vi "Connect Merge Error Terminals.vi"(8 "error in (no error)":errorcluster, 11 "DVR VI Path":path=path "D:/GitHub/LabVIEW/SLL/Tools/Class DVR API Generator/Test/Test VI.vi") -> (0 "error out":errorcluster)   [LabVIEW 2016, in "SLL Scripting.lvlib" / "SLL Class DVR API Generator.lvlib"]
uses:
  SLL Class DVR API Generator.lvlib
  <vilib>/Utility/traverseref.llb/TRef TravTarget.ctl
  <vilib>/Utility/traverseref.llb/VI Scripting - Traverse.lvlib
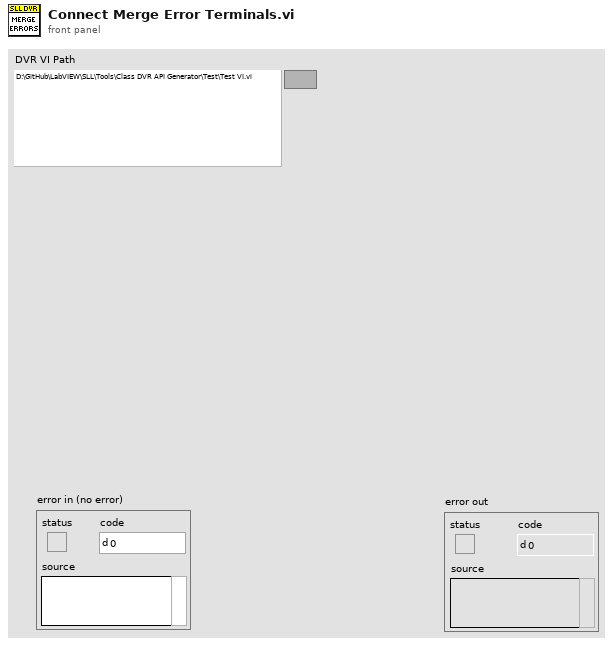
[diagram p1: front panel]
types:
  T1 = typedef "TRef TravTarget.ctl" = enum16{"FP", "BD", "Other"}
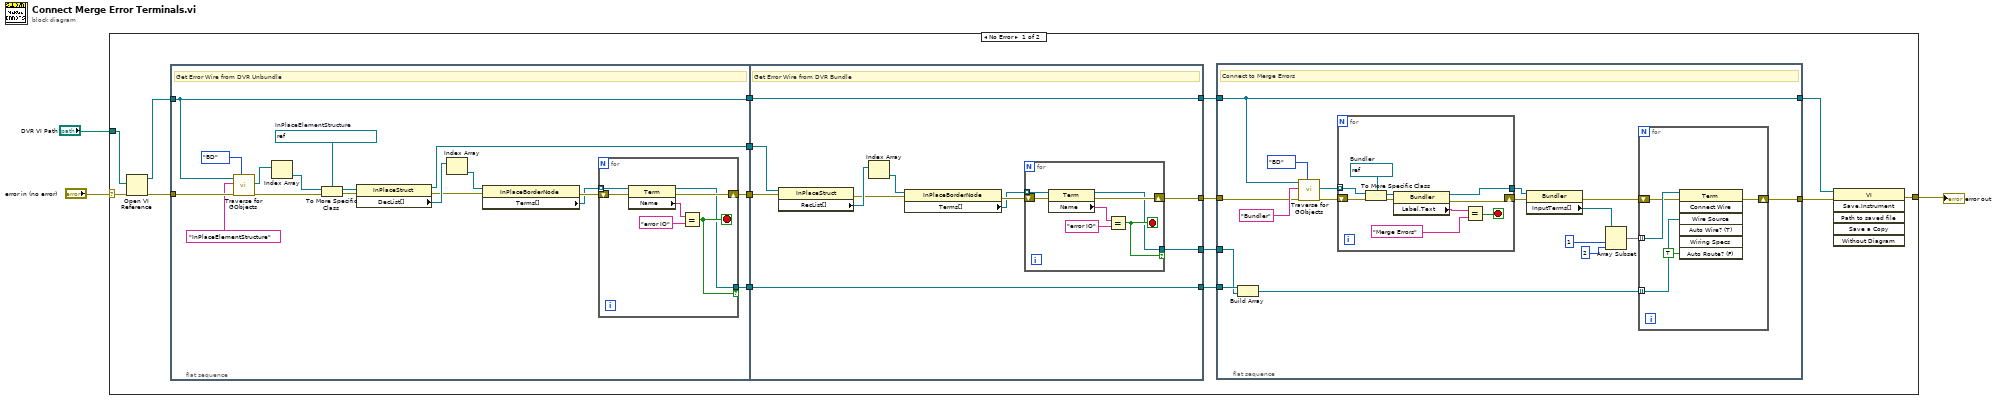
[diagram p0: block diagram]
diagram:
  n1 = case shown="No Error" "error in (no error)" {
    selector: "error in (no error)" -> [w18 w94]
    tunnel: [w16 w94] -> w2
    tunnel: "DVR VI Path" -> [w17 _]
    frame No Error {
      n2 = Open VI Reference(vi path=w17, error in (no error)=w18) -> (vi reference=w15:refnum<vi>, error out=w14:errorcluster)  [unwired: 4 in]
      n3 = flat-sequence {
        tunnel: w14 -> [w68]
        tunnel: w15 -> [w67]
        tunnel: [w67] -> w10
        tunnel: [w61] -> w9
        tunnel: [w60] -> w8
        tunnel: [w59] -> w7
        tunnel: [w86] -> w13
        tunnel: w10 -> [w86]
        tunnel: w9 -> [w82]
        tunnel: w8 -> [w81]
        tunnel: w7 -> [w80]
        tunnel: [w80] -> w6
        tunnel: [w77] -> w5
        tunnel: [w76] -> w4
        frame #0 {
          w53 = refnum<vi> refnum  # InPlaceElementStructure
          # "Get Error Wire from DVR Unbundle"
          n4 = call <vilib>:"Traverse for GObjects.vi"("Traverse Target"=TRef_TravTarget."BD", "error in (no error)"=w68, "Class Name"="InPlaceElementStructure", "VI Refnum"=w67) -> ("error out"=w55:errorcluster, "References"=w56:refnum<vi>[])  [unwired: 4 in, 2 out]
          n5 = Index Array(array=w56) -> (element=w54:refnum<vi>)  [unwired: 1 in]
          n6 = To More Specific Class(target class=w53, reference=w54, error in=w55) -> (specific class reference=w52:refnum<vi>, error out=w51:errorcluster)
          n7 = property class="InPlaceStruct"(reference=w52, error in=w51) -> (reference out=w60:refnum<vi>, error out=w64:errorcluster, "DecList[]"=w66:refnum<vi>[])
          n8 = Index Array(array=w66) -> (element=w65:refnum<vi>)  [unwired: 1 in]
          n9 = property class="InPlaceBorderNode"(reference=w65, error in=w64) -> (error out=w63:errorcluster, "Terms[]"=w62:refnum<vi>[])  [unwired: 1 out]
          n10 = for {
            tunnel: w62 -> [w75] mode=indexing
            shift-right: [w70] -> w61
            shift-left: w63 -> [w74]
            tunnel: [w69] -> w59 if=w71
            stop <- w71 stop-if-true
            n11 = property class="Term"(reference=w75, error in=w74) -> (reference out=w69:refnum<vi>, error out=w70:errorcluster, "Name"=w73:string)
            n12 = Equal?(x=w73, y="error IO") -> (x = y?=w71:bool)
          }
        }
        frame #1 {
          # "Get Error Wire from DVR Bundle"
          n13 = property class="InPlaceStruct"(reference=w81, error in=w82) -> (error out=w83:errorcluster, "RecList[]"=w85:refnum<vi>[])  [unwired: 1 out]
          n14 = Index Array(array=w85) -> (element=w84:refnum<vi>)  [unwired: 1 in]
          n15 = property class="InPlaceBorderNode"(reference=w84, error in=w83) -> (error out=w79:errorcluster, "Terms[]"=w78:refnum<vi>[])  [unwired: 1 out]
          n16 = for {
            tunnel: w78 -> [w93] mode=indexing
            shift-right: [w88] -> w77
            shift-left: w79 -> [w92]
            tunnel: [w87] -> w76 if=w89
            stop <- w89 stop-if-true
            n17 = property class="Term"(reference=w93, error in=w92) -> (reference out=w87:refnum<vi>, error out=w88:errorcluster, "Name"=w91:string)
            n18 = Equal?(x=w91, y="error IO") -> (x = y?=w89:bool)
          }
        }
      }
      n19 = flat-sequence {
        tunnel: w13 -> [w22]
        tunnel: [w29] -> w12
        tunnel: [w22] -> w11
        tunnel: w6 -> [w28]
        tunnel: w5 -> [w23]
        tunnel: w4 -> [w27]
        frame #0 {
          # "Connect to Merge Errors"
          n20 = Build Array(w28, w27) -> (w30:refnum<vi>[])
          n21 = call <vilib>:"Traverse for GObjects.vi"("Traverse Target"=TRef_TravTarget."BD", "error in (no error)"=w23, "Class Name"="Bundler", "VI Refnum"=w22) -> ("error out"=w24:errorcluster, "References"=w20:refnum<vi>[])  [unwired: 4 in, 2 out]
          n22 = for {
            shift-right: [w45] -> w21
            shift-left: w24 -> [w50]
            tunnel: w20 -> [w48] mode=indexing
            tunnel: [w44] -> w19
            stop <- w42 stop-if-true
            w49 = refnum<vi> refnum  # Bundler
            n23 = To More Specific Class(target class=w49, reference=w48, error in=w50) -> (specific class reference=w46:refnum<vi>, error out=w47:errorcluster)
            n24 = property class="Bundler"(reference=w46, error in=w47) -> (reference out=w44:refnum<vi>, error out=w45:errorcluster, "Label.Text"=w43:string)
            n25 = Equal?(x=w43, y="Merge Errors") -> (x = y?=w42:bool)
          }
          n26 = property class="Bundler"(reference=w19, error in=w21) -> (error out=w31:errorcluster, "InputTerms[]"=w35:refnum<vi>[])  [unwired: 1 out]
          n27 = Array Subset(array=w35, index=1, length=2) -> (w32:refnum<vi>[])
          n28 = for {
            tunnel: w32 -> [w40] mode=indexing
            shift-right: [w37] -> w29
            shift-left: w31 -> [w39]
            tunnel: w30 -> [w38] mode=indexing
            n29 = invoke class="Term" method="Connect Wire"(reference=w40, error in=w39, "Wire Source"=w38, "Auto Route? (F)"=TRUE) -> (error out=w37:errorcluster)  [unwired: 3 in, 6 out]
          }
        }
      }
      n30 = invoke class="VI" method="Save.Instrument"(reference=w11, error in=w12) -> (error out=w16:errorcluster)  [unwired: 4 in, 5 out]
    }
    frame Error {
    }
  }
  "error out" <- w2
